vi "2b_control_val.vi"(8 "down/back":string="x", 9 "up/fwd":string="z", 10 "down/back":bool, 11 "Up/fwd":bool) -> (3 "control_val":string)   [LabVIEW 2012]
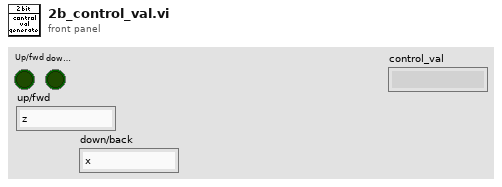
[diagram p1: front panel]
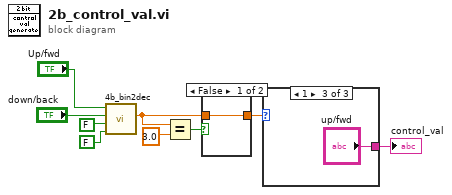
[diagram p0: block diagram]
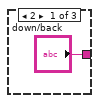
[diagram p2: hidden frame]
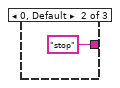
[diagram p3: hidden frame]
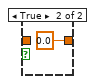
[diagram p4: hidden frame]
diagram:
  n1 = call "4b_bin2dec.vi"("Right"=FALSE, "Left"=FALSE, "Down"="down/back", "Up"="Up/fwd") -> ("Out"=w5:dbl)  [unwired: 7 in]
  n2 = Equal?(x=w5, y=3.0) -> (x = y?=w6:bool)
  n3 = case shown="False" w6 {
    tunnel: [w10 0.0 ("Out")] -> w4
    tunnel: w5 -> [w10 _]
    frame False {
    }
    frame True {
    }
  }
  n4 = case shown="1" w4 {
    tunnel: ["down/back" "stop" "up/fwd"] -> w1
    frame 2 {
    }
    frame 0, Default {
    }
    frame 1 {
    }
  }
  "control_val" <- w1
